vi "DH_Jacobian.vi"(2 "Joints":T2(array[cluster])=[{"Theta"=5.729578018188477, "d"=0.2, "a"=0.0, "alpha (degrees)"=-90.0}, {"Theta"=11.459156036376953, "d"=0.0, "a"=0.4, "alpha (degrees)"=0.0}, {"Theta"=17.18873405456543, "d"=0.0, "a"=0.0, "alpha (degrees)"=-90.0}, {"Theta"=22.918312072753906, "d"=0.4, "a"=0.0, "alpha (degrees)"=90.0}, {"Theta"=28.647890090942383, "d"=0.0, "a"=0.0, "alpha (degrees)"=-90.0}, {"Theta"=34.37746810913086, "d"=0.1, "a"=0.0, "alpha (degrees)"=0.0}] {"alpha (degrees)" format="%.2f"; "a" format="%.2f"; "d" scale=0.0..0.5; "Theta" scale=-180.0..180.0}) -> (0 "Jacobian":dbl[][](array[numeric])=[[0.4863453905069739, 2.4914071031242934e-17, -0.3570687357077486, -0.01042603129352488, -0.031186231060327, 0.0], [0.030499600323496263, -5.289101414408914e-19, 0.007580345872437841, -0.001961685850492488, -0.005867773314590696, -0.0], [-0.0, 0.04921459245874227, 0.19367959050162675, -0.02384233267087602, 0.04484823501248461, -0.0], [0.0, -0.09983341780827708, -0.4770304128923103, 0.24808677199962254, -0.8228592321708784, -0.8228592321708784], [0.0, 0.9950041651614921, -0.04786269061477082, 0.9505772695864821, 0.10507318129704712, 0.10507318129704712], [1.0, 6.123233995736766e-17, -0.8775825590922524, -0.18669710256004374, -0.5584463363683838, -0.5584463363683838]] format="%#.3f", 1 "end effector pose":T1=[[0.2818556107229001, -0.49341675968208987, -0.8228592321708784, 0.11697004227643469], [-0.7778734424176673, -0.6195744782940995, 0.10507318129704712, 0.030499600323496263], [-0.5616674481268332, 0.6104648778688426, -0.5584463363683838, -0.2863453905069739], [0.0, 0.0, 0.0, 1.0]] format="%#_2g")   [LabVIEW 2024]
uses:
  <vilib>/Analysis/Matrix/Datatypes/RealMatrix.ctl
  <vilib>/Analysis/Matrix/NI_Matrix.lvlib
panel:
  # "[[-6.12323400e-17 -5.00000000e-01 -5.00000000e-01  0.00000000e+00\n  -1.00000000e-01 -6.16297582e-33]\n [ 4.00000000e-01  2.44929360e-17  0.00000000e+00  0.00000000e+00\n   0.00000000e+00  0.00000000e+00]\n [ 0.00000000e+00 -4.00000000e-01  0.00000000e+00  0.00000000e+00\n   0.00000000e+00  0.00000000e+00]\n [ 0.00000000e+00  0.00000000e+00  0.00000000e+00  0.00000000e+00\n   0.00000000e+00  0.00000000e+00]\n [ 0.00000000e+00  1.00000000e+00  1.00000000e+00  1.22464680e-16\n   1.00000000e+00  1.22464680e-16]\n [ 1.00000000e+00  6.12323400e-17  6.12323400e-17 -1.00000000e+00\n   6.12323400e-17 -1.00000000e+00]]"
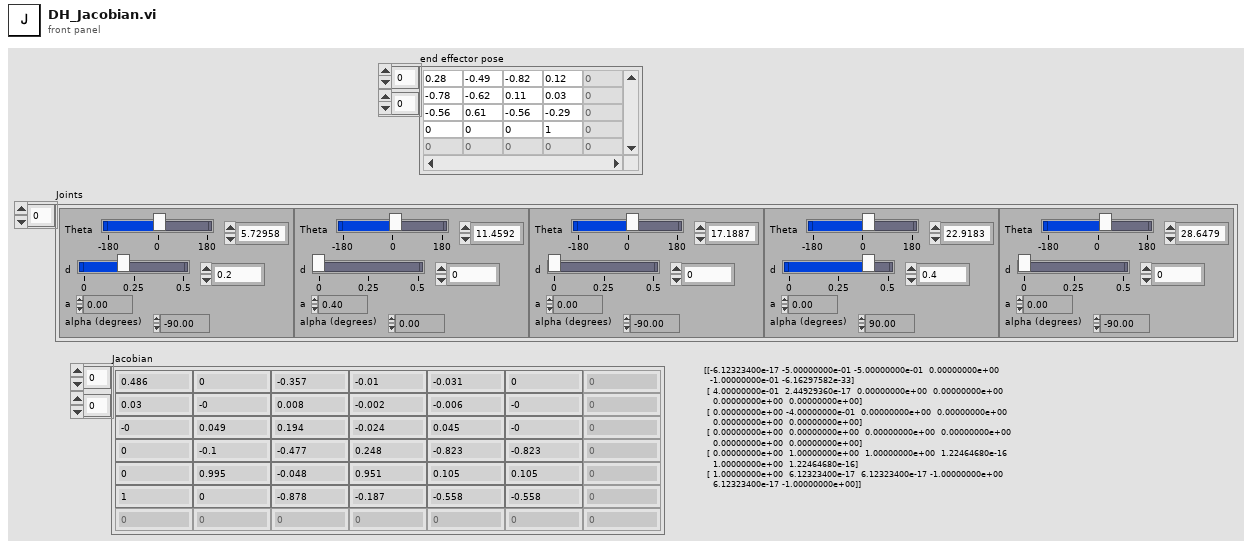
[diagram p1: front panel]
types:
  T1 = typedef "NI_Matrix.lvlib/RealMatrix.ctl" = dbl[][]
  T2 = cluster{"Theta":dbl, "d":dbl, "a":dbl, "alpha (degrees)":dbl}[]
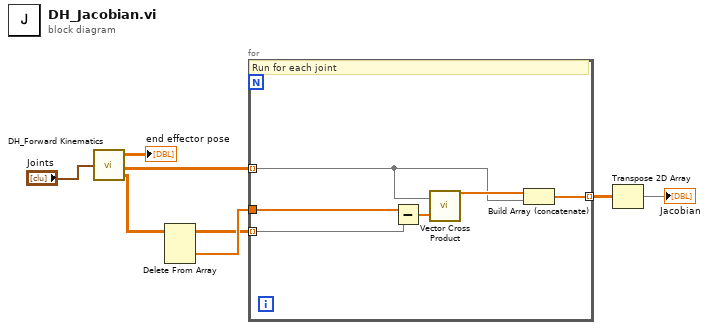
[diagram p0: block diagram]
diagram:
  n1 = call <userlib>:"DH_Forward Kinematics.vi"("Joints"="Joints") -> ("end effector pose"=→"end effector pose":T1, "z_i"=w4:dbl[][], "positions"=w2:dbl[][])  [unwired: 3 in, 1 out]
  n2 = Delete From Array "Delete From Array"(array=w2) -> (deleted portion=w3:dbl[], array with subset deleted=w1:dbl[][])  [unwired: 3 in]
  n3 = for {
    tunnel: [w12] -> w8 mode=indexing
    tunnel: w3 -> [w11]
    tunnel: w4 -> [w10] mode=indexing
    tunnel: w1 -> [w9] mode=indexing
    # "Run for each joint"
    n4 = Subtract(x=w11, y=w9) -> (x-y=w14:dbl[])
    n5 = call <userlib>:"Vector Cross Product.vi"("B"=w14, "A"=w10) -> ("A x B"=w13:dbl[])  [unwired: 1 in]
    n6 = Build Array (concatenate)(w13, w10) -> (w12:dbl[])
  }
  n7 = Transpose 2D Array(2D array=w8) -> (transposed array=→"Jacobian":dbl[][])
